vi "信号定位3-matlab.vi"() -> ()   [LabVIEW 2013]
panel:
  out "y":dbl
  out "x":dbl
  in  "速度m/s":dbl=1.0
  in  "y3":dbl
  in  "x3":dbl
  in  "y2":dbl
  in  "x2":dbl
  in  "y1":dbl
  in  "x1":dbl
  in  "signal 3":dbl
  in  "signal 2":dbl
  in  "signal 1":dbl
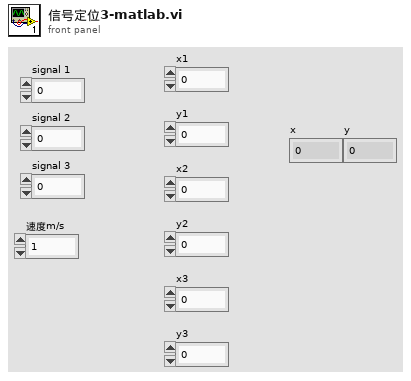
[diagram p1: front panel]
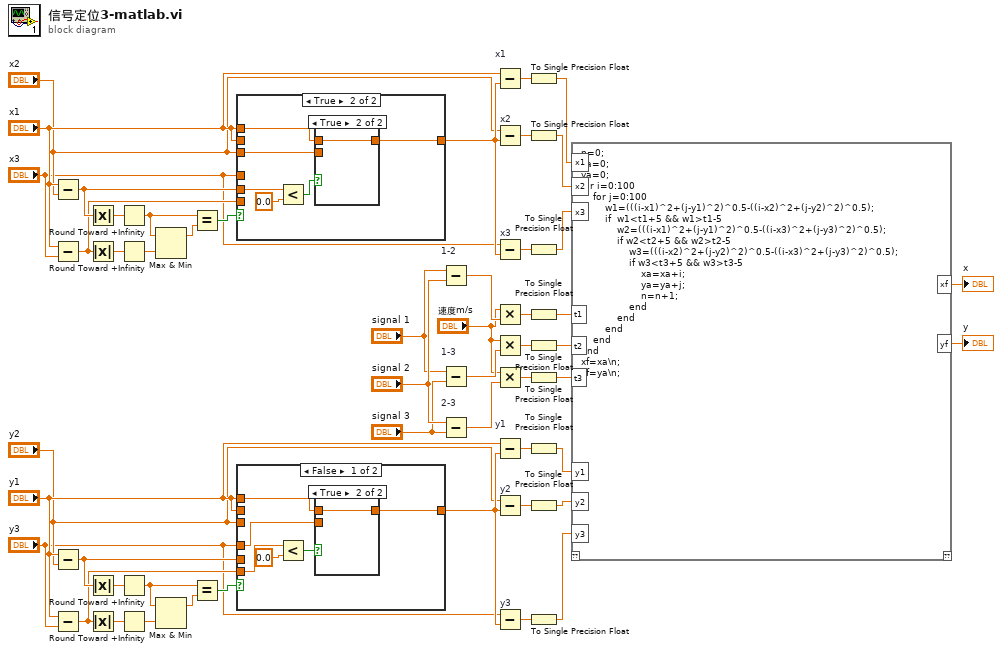
[diagram p0: block diagram]
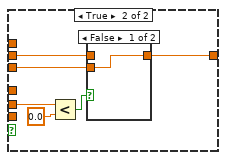
[diagram p3: hidden frame]
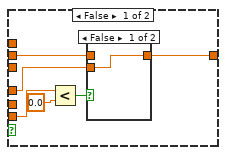
[diagram p5: hidden frame]
diagram:
  n1 = Subtract(x="x1", y="x2") -> (x-y=w30:dbl)
  n2 = Subtract(x="x1", y="x3") -> (x-y=w29:dbl)
  n3 = Subtract(x="y1", y="y2") -> (x-y=w32:dbl)
  n4 = Subtract(x="y1", y="y3") -> (x-y=w31:dbl)
  n5 = Absolute Value(x=w30) -> (abs(x)=w42:dbl)
  n6 = Absolute Value(x=w29) -> (abs(x)=w41:dbl)
  n7 = Absolute Value(x=w32) -> (abs(x)=w34:dbl)
  n8 = Absolute Value(x=w31) -> (abs(x)=w33:dbl)
  n9 = Round Toward +Infinity(x=w42) -> (ceil(x): smallest int >= x=w38:dbl)
  n10 = Round Toward +Infinity(x=w41) -> (ceil(x): smallest int >= x=w48:dbl)
  n11 = Round Toward +Infinity(x=w34) -> (ceil(x): smallest int >= x=w35:dbl)
  n12 = Round Toward +Infinity(x=w33) -> (ceil(x): smallest int >= x=w47:dbl)
  n13 = Max & Min(x=w38, y=w48) -> (max(x,y)=w39:dbl)  [unwired: 1 out]
  n14 = Max & Min(x=w35, y=w47) -> (max(x,y)=w36:dbl)  [unwired: 1 out]
  n15 = Equal?(x=w38, y=w39) -> (x = y?=w40:bool)
  n16 = Equal?(x=w35, y=w36) -> (x = y?=w37:bool)
  n17 = case shown="True" w40 {
    tunnel: w30 -> [_ w63]
    tunnel: "x1" -> [_ w62]
    tunnel: [w53 w61] -> w28
    tunnel: "x2" -> [_ w60]
    tunnel: w29 -> [w55 _]
    tunnel: "x1" -> [w54 _]
    tunnel: "x3" -> [w52 _]
    frame False {
      n18 = Less?(x=w55, y=0.0) -> (x < y?=w56:bool)
      n19 = case shown="False" w56 {
        tunnel: w54 -> [_ w59]
        tunnel: [w58 w59] -> w53
        tunnel: w52 -> [w58 _]
        frame False {
        }
        frame True {
        }
      }
    }
    frame True {
      n20 = Less?(x=w63, y=0.0) -> (x < y?=w65:bool)
      n21 = case shown="True" w65 {
        tunnel: w62 -> [_ w67]
        tunnel: [w66 w67] -> w61
        tunnel: w60 -> [w66 _]
        frame False {
        }
        frame True {
        }
      }
    }
  }
  n22 = case shown="False" w37 {
    tunnel: w32 -> [_ w79]
    tunnel: "y1" -> [_ w78]
    tunnel: [w69 w77] -> w24
    tunnel: "y2" -> [_ w76]
    tunnel: w31 -> [w71 _]
    tunnel: "y1" -> [w70 _]
    tunnel: "y3" -> [w68 _]
    frame False {
      n23 = Less?(x=w71, y=0.0) -> (x < y?=w72:bool)
      n24 = case shown="True" w72 {
        tunnel: w70 -> [_ w75]
        tunnel: [w74 w75] -> w69
        tunnel: w68 -> [w74 _]
        frame False {
        }
        frame True {
        }
      }
    }
    frame True {
      n25 = Less?(x=w79, y=0.0) -> (x < y?=w81:bool)
      n26 = case shown="False" w81 {
        tunnel: w78 -> [_ w83]
        tunnel: [w82 w83] -> w77
        tunnel: w76 -> [w82 _]
        frame False {
        }
        frame True {
        }
      }
    }
  }
  n27 = Subtract "1-2"(x="signal 1", y="signal 2") -> (x-y=w46:dbl)
  n28 = Subtract "1-3"(x="signal 1", y="signal 3") -> (x-y=w45:dbl)
  n29 = Subtract "2-3"(x="signal 2", y="signal 3") -> (x-y=w44:dbl)
  n30 = Subtract "x1"(x="x1", y=w28) -> (x-y=w12:dbl)
  n31 = Subtract "x2"(x="x2", y=w28) -> (x-y=w20:dbl)
  n32 = Subtract "x3"(x="x3", y=w28) -> (x-y=w19:dbl)
  n33 = Multiply(x="速度m/s", y=w46) -> (x*y=w15:dbl)
  n34 = Multiply(x="速度m/s", y=w45) -> (x*y=w14:dbl)
  n35 = Multiply(x="速度m/s", y=w44) -> (x*y=w13:dbl)
  n36 = Subtract "y1"(x="y1", y=w24) -> (x-y=w18:dbl)
  n37 = Subtract "y2"(x="y2", y=w24) -> (x-y=w17:dbl)
  n38 = Subtract "y3"(x="y3", y=w24) -> (x-y=w16:dbl)
  n39 = To Single Precision Float(number=w12) -> (single precision float=w11:sgl)
  n40 = To Single Precision Float(number=w20) -> (single precision float=w10:sgl)
  n41 = To Single Precision Float(number=w19) -> (single precision float=w9:sgl)
  n42 = To Single Precision Float(number=w15) -> (single precision float=w8:sgl)
  n43 = To Single Precision Float(number=w14) -> (single precision float=w7:sgl)
  n44 = To Single Precision Float(number=w13) -> (single precision float=w6:sgl)
  n45 = To Single Precision Float(number=w18) -> (single precision float=w5:sgl)
  n46 = To Single Precision Float(number=w17) -> (single precision float=w4:sgl)
  n47 = To Single Precision Float(number=w16) -> (single precision float=w3:sgl)
  n48 = script code="n=0;\nxa=0;\nya=0;\nfor i=0:100\n    for j=0:100\n        w1=(((i-x1)^2+(j-y1)^2)^0.5-((i-x2)^2+(j-y2)^2)^0.5);\n        if  w1<t1+5 && w1>t1-5\n            w2=(((i-x1)^2+(j-y1)^2)^0.5-((i-x3)^2+(j-y3)^2)^0.5);\n            if w2<t2+5 && w2>t2-5\n                w3=(((i-x2)^2+(j-y2)^2)^0.5-((i-x3)^2+(j-y3)^2)^0.5);\n                if w3<t3+5 && w3>t3-5\n                    xa=xa+i;\n                    ya=ya+j;\n                    n=n+1;\n                end\n            end\n        end\n    end\nend\nxf=xa\\n;\nyf=ya\\n;"("x1"=w11, "x2"=w10, "x3"=w9, "y1"=w5, "y2"=w4, "y3"=w3, "t1"=w8, "t2"=w7, "t3"=w6) -> ("xf"=→"x":dbl, "yf"=→"y":dbl)  [unwired: 1 in, 1 out]
